vi "Teleop.vi"(10 "Match Info":T1={"Autonomous Elapsed Seconds"=0.0, "TeleOp Elapsed Seconds"=0.0, "Disabled Elapsed Seconds"=0.0, "Visited Autonomous"=FALSE, "Visited TeleOp"=FALSE, "Visited Disabled"=FALSE, "Autonomous Settings"={"Autonomous Style"=enum."Independent", "VI Refnum"=refnum}}, 11 "Call Context":T2) -> ()   [LabVIEW 2020]
doc: "This VI is called for each enabled TeleOp packet received from the DS. It is typically used to read from joysticks and other inputs and update I/O or setpoints for timed control loops. It should complete and return within 20 milliseconds or risk missing DS packets."
uses:
  <vilib>/Rock Robotics/WPI/DriverStation/WPI_DriverStationDerivedRobotMode.ctl
  <vilib>/Rock Robotics/WPI/DriverStation/WPI_DriverStationMatch Info.ctl
  Framework/Robot Global Data.vi
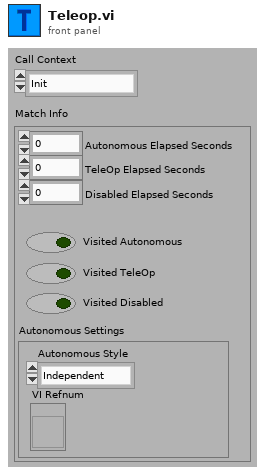
[diagram p1: front panel]
types:
  T1 = typedef "WPI_DriverStationMatch Info.ctl" = cluster{"Autonomous Elapsed Seconds":dbl, "TeleOp Elapsed Seconds":dbl, "Disabled Elapsed Seconds":dbl, "Visited Autonomous":bool, "Visited TeleOp":bool, "Visited Disabled":bool, "Autonomous Settings":cluster{"Autonomous Style":enum16{"Iterative", "Independent"}, "VI Refnum":refnum<vi>}}
  T2 = typedef "WPI_DriverStationDerivedRobotMode.ctl" = enum16{"Init", "Execute", "Stop"}
  T3 = typedef "Command Status Info.ctl" = cluster{"Name":string, "Status":T4, "notifier out":T5}
  T4 = typedef "Completion Status.ctl" = enum16{"Successful", "Aborted", "Incomplete"}
  T5 = typedef "Completion Notifier.ctl" = refnum<notifier>
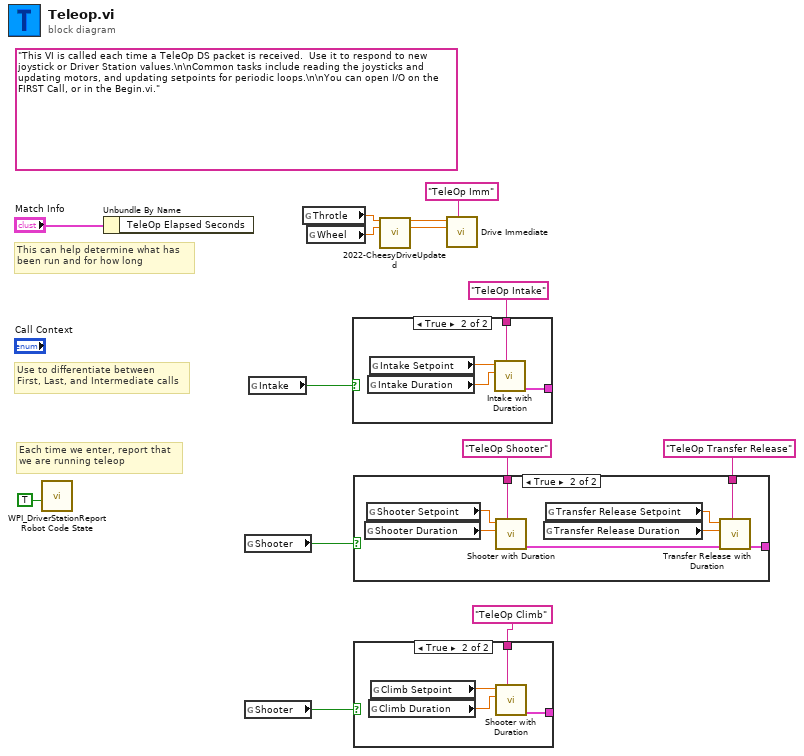
[diagram p0: block diagram]
diagram:
  (unwired) "This VI is called each time a TeleOp DS packet is received.  Use it to respond to new joystick or Driver Station values.\n\nCommon tasks include reading the joysticks and updating motors, and updating setpoints for periodic loops.\n\nYou can open I/O on the FIRST Call, or in the Begin.vi."
  # "Each time we enter, report that\nwe are running teleop"
  # "Use to differentiate between\nFirst, Last, and Intermediate calls"
  # "This can help determine what has\nbeen run and for how long"
  n1 = call <vilib>:"WPI_DriverStationReport Robot Code State.vi"("TeleOp"=TRUE ("Autonomous")) -> ()  [unwired: 10 in, 1 out]
  n2 = Unbundle By Name("Match Info") -> ()  [unwired: 1 out]
  n3 = global read "Robot Global Data.vi" "Shooter"() -> (w5:bool)
  n4 = global read "Robot Global Data.vi" "Shooter"() -> (w2:bool)
  n5 = global read "Robot Global Data.vi" "Intake"() -> (w6:bool)
  n6 = global read "Robot Global Data.vi" "Throtle"() -> (w8:dbl)
  n7 = global read "Robot Global Data.vi" "Wheel"() -> (w7:dbl)
  n8 = case shown="True" w6 {
    tunnel: [_ w18] -> _
    tunnel: "TeleOp Intake" ("Description") -> [_ w17]
    frame False {
    }
    frame True {
      n9 = global read "Robot Global Data.vi" "Intake Duration"() -> (w15:dbl)
      n10 = global read "Robot Global Data.vi" "Intake Setpoint"() -> (w16:dbl)
      n11 = call "Intake with Duration.vi"("Description"=w17, "Duration (s)"=w15, "Setpoint"=w16) -> ("Command Info Out"=w18:T3)  [unwired: 8 in]
    }
  }
  n12 = case shown="True" w5 {
    tunnel: "TeleOp Shooter" ("Description") -> [_ w26]
    tunnel: [_ w22] -> _
    tunnel: "TeleOp Transfer Release" ("Description") -> [_ w21]
    frame False {
    }
    frame True {
      n13 = global read "Robot Global Data.vi" "Shooter Duration"() -> (w24:dbl)
      n14 = global read "Robot Global Data.vi" "Shooter Setpoint"() -> (w25:dbl)
      n15 = call "Shooter with Duration.vi"("Description"=w26, "Duration (s)"=w24, "Setpoint"=w25) -> ("Command Info Out"=w23:T3)  [unwired: 8 in]
      n16 = global read "Robot Global Data.vi" "Transfer Release Duration"() -> (w20:dbl)
      n17 = global read "Robot Global Data.vi" "Transfer Release Setpoint"() -> (w19:dbl)
      n18 = call "Transfer Release with Duration.vi"("Description"=w21, "Command Info In"=w23, "Duration (s)"=w20, "Setpoint"=w19) -> ("Command Info Out"=w22:T3)  [unwired: 7 in]
    }
  }
  n19 = case shown="True" w2 {
    tunnel: [_ w30] -> _
    tunnel: "TeleOp Climb" ("Description") -> [_ w29]
    frame False {
    }
    frame True {
      n20 = global read "Robot Global Data.vi" "Climb Duration"() -> (w27:dbl)
      n21 = global read "Robot Global Data.vi" "Climb Setpoint"() -> (w28:dbl)
      n22 = call "Shooter with Duration.vi"("Description"=w29, "Duration (s)"=w27, "Setpoint"=w28) -> ("Command Info Out"=w30:T3)  [unwired: 8 in]
    }
  }
  n23 = call "2022-CheesyDriveUpdated.vi"("Throttle"=w8, "Wheel"=w7) -> ("Left PWM"=w10:dbl, "Right PWM"=w9:dbl)  [unwired: 11 in, 1 out]
  n24 = call "Drive Immediate.vi"("Description"="TeleOp Imm", "Right Setpoint"=w9, "Left Setpoint"=w10) -> ()  [unwired: 8 in, 1 out]
